vi "Reports - Exact Match.vi"(1 "BOM Item":T6, 2 "Inventory Item":T1) -> (0 "Line Item Report":string)   [LabVIEW 2013]
uses:
  BOM Item.ctl
  Controls/Components.ctl
  Controls/Component Sub Type.ctl
  Controls/Display Component Line.ctl
  Controls/Add Button.ctl
  Controls/Subtract Button.ctl
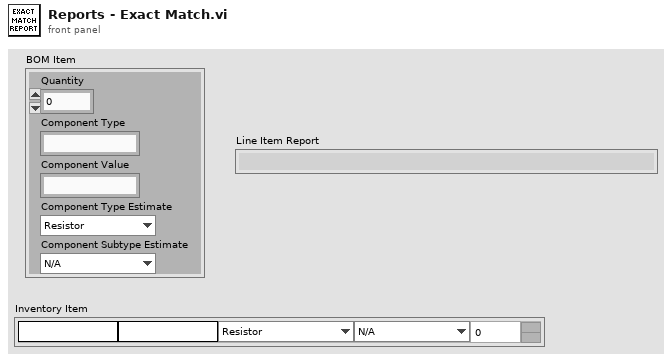
[diagram p1: front panel]
types:
  T1 = typedef "Display Component Line.ctl" = cluster{"Part Number":string, "Code (Value)":string, "Component Type":T2, "Component Subtype":T3, "Quantity":u32, "Add":T4, "Subtract":T5}
  T2 = typedef "Components.ctl" = enum16{"Resistor", "Capacitor", "Diode", "Voltage Regulator", "Transistors", "ICs", "Misc"}
  T3 = typedef "Component Sub Type.ctl" = enum16{"N/A", "Carbon", "Variable - Trimmer", "Variable - Pot", "Ceramic", "Electrolitic", "Zenner", "TO-92", "TO-220", "NPN", "PNP", "CMOS", "Processor"}
  T4 = typedef "Add Button.ctl" = bool
  T5 = typedef "Subtract Button.ctl" = bool
  T6 = typedef "BOM Item.ctl" = cluster{"Quantity":i32, "Component Type":string, "Component Value":string, "Component Type Estimate":T2, "Component Subtype Estimate":T3}
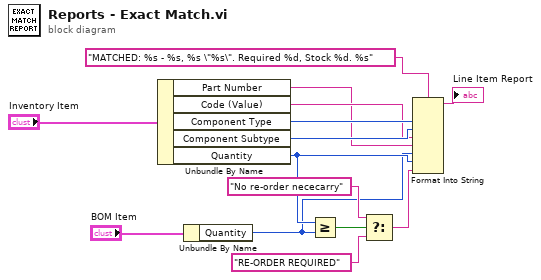
[diagram p0: block diagram]
diagram:
  n1 = Unbundle By Name("Inventory Item") -> ("Part Number"=w1:string, "Code (Value)"=w7:string, "Component Type"=w9:T2, "Component Subtype"=w8:T3, "Quantity"=w5:u32)
  n2 = Unbundle By Name("BOM Item") -> ("Quantity"=w2:i32)
  n3 = Greater Or Equal?(x=w5, y=w2) -> (x >= y?=w4:bool)
  n4 = Select(t="No re-order nececarry", s=w4, f="RE-ORDER REQUIRED") -> (s? t:f=w6:string)
  n5 = Format Into String(format string="MATCHED: %s - %s, %s \"%s\". Required %d, Stock %d. %s", w9, w8, w7, w1, w2, w5, w6) -> (resulting string=→"Line Item Report":string)  [unwired: 2 in, 1 out]
